vi "MododeJogo.vi"() -> ()   [LabVIEW 2011]
doc: "VI resposável por todas as configurações pré-jogo, como: número e nomes dos jogadores."
panel:
  in  "NívelAsiático":bool
  in  "NívelDifícil":bool
  in  "NívelMédio":bool
  in  "NívelFácil":bool
  in  "BotaoVoltar":bool
  in  "BotaoComecar":bool
  in  "Jogador 2":string
  in  "Jogador 1":string
  in  "2Jogadores":bool=TRUE
  in  "1Jogador":bool
  # "Modo de Jogo"
  # "Dificuldade"
  # "Fácil"
  # "1 Jogador"
  # "Médio"
  # "Difícil"
  # "2 Jogadores"
  # "Asiático"
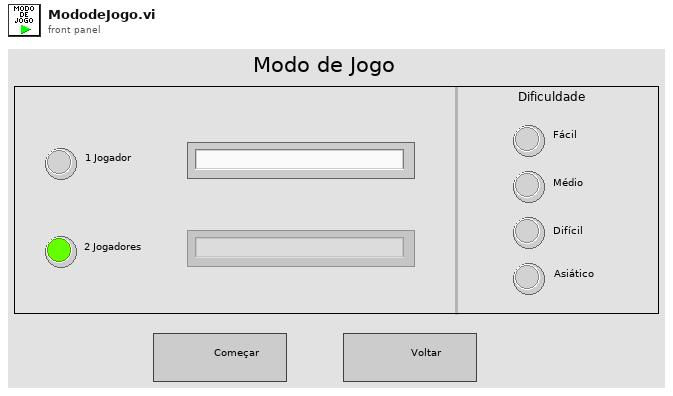
[diagram p1: front panel]
types:
  T1 = enum8{"Enabled", "Disabled", "Disabled and Grayed Out"}
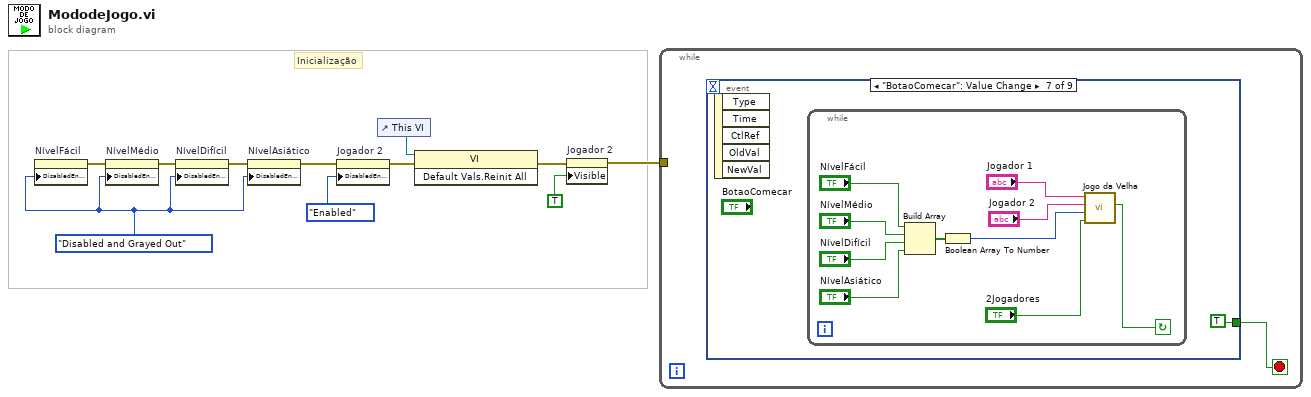
[diagram p0: block diagram]
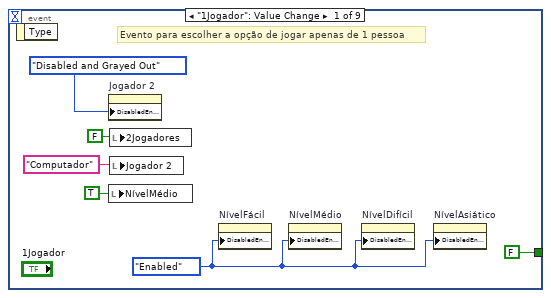
[diagram p2: hidden frame]
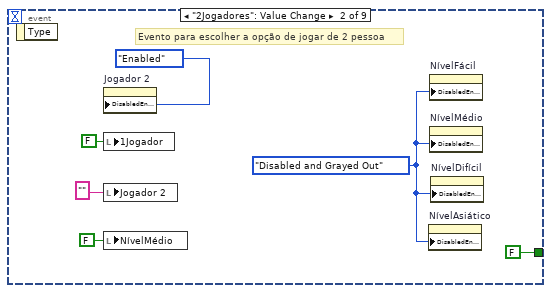
[diagram p3: hidden frame]
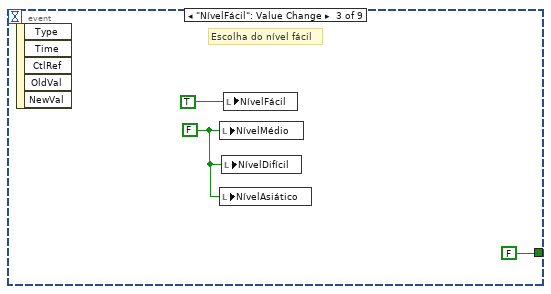
[diagram p4: hidden frame]
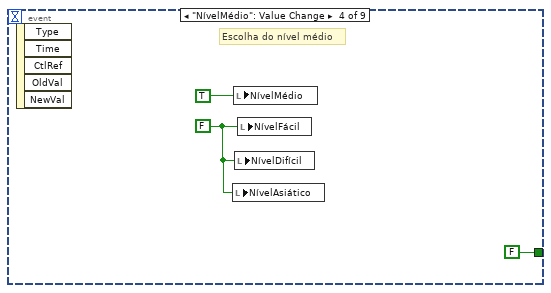
[diagram p5: hidden frame]
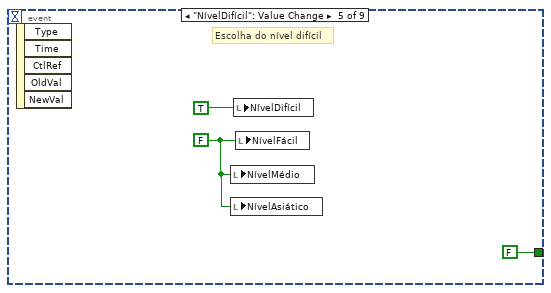
[diagram p6: hidden frame]
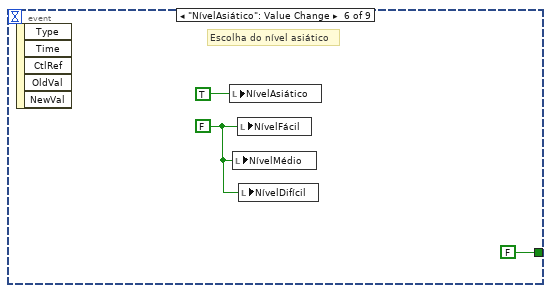
[diagram p7: hidden frame]
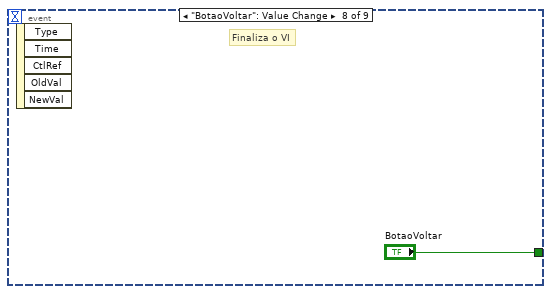
[diagram p8: hidden frame]
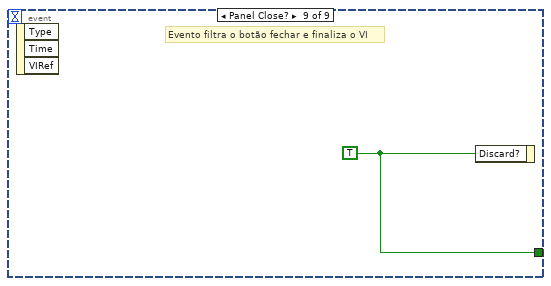
[diagram p9: hidden frame]
diagram:
  w5 = T1."Disabled and Grayed Out" ("Disabled")
  # "Inicialização"
  n1 = property on="NívelFácil" class="Bool (strict)"("DisabledEnum"=w5) -> (error out=w1:errorcluster)  [unwired: 2 in, 1 out]
  n2 = property on="NívelMédio" class="Bool (strict)"(error in=w1, "DisabledEnum"=w5) -> (error out=w2:errorcluster)  [unwired: 1 in, 1 out]
  n3 = property on="NívelDifícil" class="Bool (strict)"(error in=w2, "DisabledEnum"=w5) -> (error out=w3:errorcluster)  [unwired: 1 in, 1 out]
  n4 = property on="NívelAsiático" class="Bool (strict)"(error in=w3, "DisabledEnum"=w5) -> (error out=w4:errorcluster)  [unwired: 1 in, 1 out]
  n5 = property on="Jogador 2" class="Str"(error in=w4, "DisabledEnum"=T1."Enabled" ("Disabled")) -> (error out=w6:errorcluster)  [unwired: 1 in, 1 out]
  n6 = control-ref of="This VI"() -> (w10:refnum<vi>)
  n7 = invoke class="VI" method="Default Vals.Reinit All"(reference=w10, error in=w6) -> (error out=w9:errorcluster)  [unwired: 1 in, 2 out]
  n8 = property on="Jogador 2" class="Str"(error in=w9, "Visible"=TRUE) -> (error out=w8:errorcluster)  [unwired: 1 in, 1 out]
  n9 = while {
    tunnel: w8 -> [_]
    stop <- w12 stop-if-true
    n10 = event shown="[6] \"BotaoComecar\": Value Change" {
      selector: _ -> [_ _ _ _ _ _ _ _ _]
      dyn-events: _ -> [_ _ _ _ _ _ _ _ _]
      timeout: _ -> [_ _ _ _ _ _ _ _ _]
      tunnel: [FALSE ("BotaoVoltar") FALSE ("BotaoVoltar") FALSE FALSE FALSE FALSE TRUE ("BotaoVoltar") "BotaoVoltar" w49] -> w12
      event "1Jogador": Value Change {
        w13 = T1."Enabled" ("Disabled")
        # "Evento para escolher a opção de jogar apenas de 1 pessoa"
        n11 = event-data() -> ()  [unwired: 1 in, 1 out]
        n12 = property on="Jogador 2" class="Str"("DisabledEnum"=T1."Disabled and Grayed Out" ("Disabled")) -> ()  [unwired: 2 in, 2 out]
        n13 = local write "NívelMédio"(TRUE ("NívelMédio")) -> ()
        n14 = local write "2Jogadores"(FALSE) -> ()
        n15 = local write "Jogador 2"("Computador" ("Jogador 2")) -> ()
        n16 = property on="NívelFácil" class="Bool (strict)"("DisabledEnum"=w13) -> ()  [unwired: 2 in, 2 out]
        n17 = property on="NívelMédio" class="Bool (strict)"("DisabledEnum"=w13) -> ()  [unwired: 2 in, 2 out]
        n18 = property on="NívelDifícil" class="Bool (strict)"("DisabledEnum"=w13) -> ()  [unwired: 2 in, 2 out]
        n19 = property on="NívelAsiático" class="Bool (strict)"("DisabledEnum"=w13) -> ()  [unwired: 2 in, 2 out]
      }
      event "2Jogadores": Value Change {
        w21 = T1."Disabled and Grayed Out" ("Disabled")
        # "Evento para escolher a opção de jogar de 2 pessoa"
        n20 = event-data() -> ()  [unwired: 1 in, 1 out]
        n21 = property on="Jogador 2" class="Str"("DisabledEnum"=T1."Enabled" ("Disabled")) -> ()  [unwired: 2 in, 2 out]
        n22 = local write "1Jogador"(FALSE ("1Player")) -> ()
        n23 = local write "Jogador 2"("" ("Jogador 2")) -> ()
        n24 = local write "NívelMédio"(FALSE ("NívelMédio")) -> ()
        n25 = property on="NívelAsiático" class="Bool (strict)"("DisabledEnum"=w21) -> ()  [unwired: 2 in, 2 out]
        n26 = property on="NívelFácil" class="Bool (strict)"("DisabledEnum"=w21) -> ()  [unwired: 2 in, 2 out]
        n27 = property on="NívelMédio" class="Bool (strict)"("DisabledEnum"=w21) -> ()  [unwired: 2 in, 2 out]
        n28 = property on="NívelDifícil" class="Bool (strict)"("DisabledEnum"=w21) -> ()  [unwired: 2 in, 2 out]
      }
      event "NívelFácil": Value Change {
        w27 = FALSE ("NívelMédio")
        # "Escolha do nível fácil"
        n29 = event-data() -> ()  [unwired: 1 in, 5 out]
        n30 = local write "NívelMédio"(w27) -> ()
        n31 = local write "NívelAsiático"(w27) -> ()
        n32 = local write "NívelDifícil"(w27) -> ()
        n33 = local write "NívelFácil"(TRUE ("NívelMédio")) -> ()
      }
      event "NívelMédio": Value Change {
        w30 = FALSE ("NívelMédio")
        # "Escolha do nível médio"
        n34 = event-data() -> ()  [unwired: 1 in, 5 out]
        n35 = local write "NívelAsiático"(w30) -> ()
        n36 = local write "NívelMédio"(TRUE ("NívelMédio")) -> ()
        n37 = local write "NívelDifícil"(w30) -> ()
        n38 = local write "NívelFácil"(w30) -> ()
      }
      event "NívelDifícil": Value Change {
        w32 = FALSE ("NívelMédio")
        # "Escolha do nível difícil"
        n39 = event-data() -> ()  [unwired: 1 in, 5 out]
        n40 = local write "NívelMédio"(w32) -> ()
        n41 = local write "NívelAsiático"(w32) -> ()
        n42 = local write "NívelDifícil"(TRUE ("NívelMédio")) -> ()
        n43 = local write "NívelFácil"(w32) -> ()
      }
      event "NívelAsiático": Value Change {
        w35 = FALSE ("NívelMédio")
        # "Escolha do nível asiático"
        n44 = event-data() -> ()  [unwired: 1 in, 5 out]
        n45 = local write "NívelAsiático"(TRUE ("NívelMédio")) -> ()
        n46 = local write "NívelMédio"(w35) -> ()
        n47 = local write "NívelFácil"(w35) -> ()
        n48 = local write "NívelDifícil"(w35) -> ()
      }
      event "BotaoComecar": Value Change {
        n49 = event-data() -> ()  [unwired: 1 in, 5 out]
        n50 = while {
          stop <- w45 continue-if-true
          n51 = Build Array("NívelFácil", "NívelMédio", "NívelDifícil", "NívelAsiático") -> (w44:bool[])
          n52 = Boolean Array To Number(Boolean array=w44) -> (number=w38:u32)
          n53 = call "Jogo da Velha.vi"("2 Jogadores?"="2Jogadores", "NívelDificuldade"=w38, "Jogador 2"="Jogador 2", "Jogador 1"="Jogador 1") -> ("JogarNovamente?"=w45:bool)  [unwired: 7 in]
        }
      }
      event "BotaoVoltar": Value Change {
        # "Finaliza o VI"
        n54 = event-data() -> ()  [unwired: 1 in, 5 out]
      }
      event Panel Close? {
        w49 = TRUE ("Discard?")
        # "Evento filtra o botão fechar e finaliza o VI"
        n55 = event-data() -> ()  [unwired: 1 in, 3 out]
        n56 = event-data("Discard?"=w49) -> ()  [unwired: 1 in, 1 out]
      }
    }
  }
